vi "Create NI 9212.vi"(8 "error in":errorcluster, 10 "channel settings":T1[](array[typedef]), 11 "module settings":T4={"conversion time"=enum."High Speed", "open thermocouple detection"=TRUE}) -> (0 "error out":errorcluster, 3 "NI 9212 out":refnum<class "NI 9212.lvclass">)   [LabVIEW 2017, in "Scan Engine Scripting.lvlib" / "NI 9212.lvclass"]
doc: "Creates and configures an instance of a 9212 module that can be used to set a slot in a scan engine custom device chassis."
uses:
  NI 9212.lvclass
  NI 9212 Settings.ctl
  NI 9212 Conversion Time.ctl
  Mode Classes/Controls/thermocouple channel settings.ctl
  Channel Classes/Thermocouple Channel/Thermocouple Type.ctl
  Channel Classes/Thermocouple Channel/Measurement Units.ctl
  Mode Classes/Thermocouple Mode/Thermocouple Mode.lvclass
  C:/Users/nitest/Documents/niveristand-scan-engine-ethercat-custom-device/Custom Device Source/Scripting/Modules/Mode Classes/Mode/Mode.lvclass
  2d70a152-dcfd-4b86-981e-c1dde91b390a.vi
  Channel Classes/Thermocouple Channel/Thermocouple Channel.lvclass
  Scan Engine Scripting.lvlib
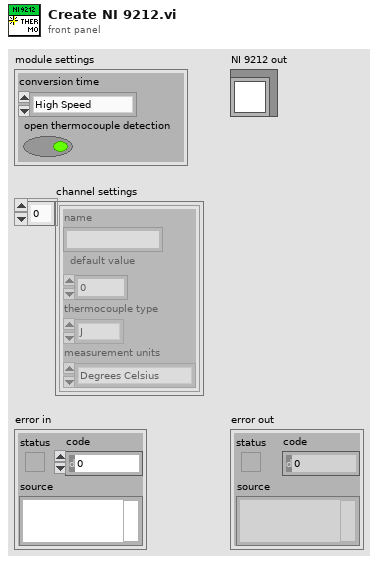
[diagram p1: front panel]
types:
  T1 = typedef "Scan Engine Scripting.lvlib/thermocouple channel settings.ctl" = cluster{"name":string, "default value":dbl, "thermocouple type":T2, "measurement units":T3}
  T2 = typedef "Scan Engine Scripting.lvlib/Thermocouple Channel.lvclass/Thermocouple Type.ctl" = enum16{"J", "K", "T", "E", "R", "S", "N", "B"}
  T3 = typedef "Scan Engine Scripting.lvlib/Thermocouple Channel.lvclass/Measurement Units.ctl" = enum16{"Raw Volts", "Degrees Kelvin", "Degrees Celsius", "Degrees Fahrenheit", "Degrees Rankine"}
  T4 = typedef "Scan Engine Scripting.lvlib/NI 9212.lvclass/NI 9212 Settings.ctl" = cluster{"conversion time":T5, "open thermocouple detection":bool}
  T5 = typedef "Scan Engine Scripting.lvlib/NI 9212.lvclass/NI 9212 Conversion Time.ctl" = enum16{"High Speed", "Best 60 Hz Rejection", "Best 50 Hz Rejection", "High Resolution"}
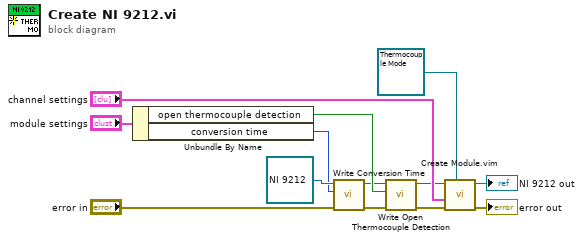
[diagram p0: block diagram]
diagram:
  n1 = Unbundle By Name("module settings") -> ("open thermocouple detection"=w9:bool, "conversion time"=w3:T5)
  n2 = call-dynamic "Write Conversion Time.vi"("error in"="error in", "conversion time"=w3, "NI 9212 in"=refnum<class "NI 9212.lvclass"> refnum ("Scan Engine Scripting.lvlib:NI 9212.lvclass")) -> ("error out"=w7:errorcluster, "NI 9212 out"=w5:refnum<class "NI 9212.lvclass">)  [unwired: 7 in]
  n3 = call-dynamic "Write Open Thermocouple Detection.vi"("error in"=w7, "open thermocouple detection"=w9, "NI 9212 in"=w5) -> ("error out"=w2:errorcluster, "NI 9212 out"=w1:refnum<class "NI 9212.lvclass">)  [unwired: 7 in]
  n4 = call "Create Module.vim"("mode in"=refnum<class "Thermocouple Mode.lvclass"> refnum ("Scan Engine Scripting.lvlib:Thermocouple Mode.lvclass"), "error in"=w2, "channel settings"="channel settings", "module in"=w1) -> ("error out"=→"error out":errorcluster, "module out"=→"NI 9212 out":refnum<class "NI 9212.lvclass">)  [unwired: 6 in]
